vi "deserialize (HW-AIM).vi"(11 "data in":string[][](array[string])) -> (3 "hw configuration":T1[](array[typedef])=[{"terminalAddress"=[0]}, {"terminalAddress"=[1]}])   [LabVIEW 2020]
uses:
  _controls/aim1553_RT_list.ctl
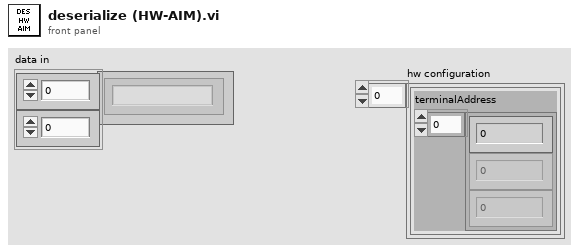
[diagram p1: front panel]
types:
  T1 = typedef "aim1553_RT_list.ctl" = cluster{"terminalAddress":i32[]}
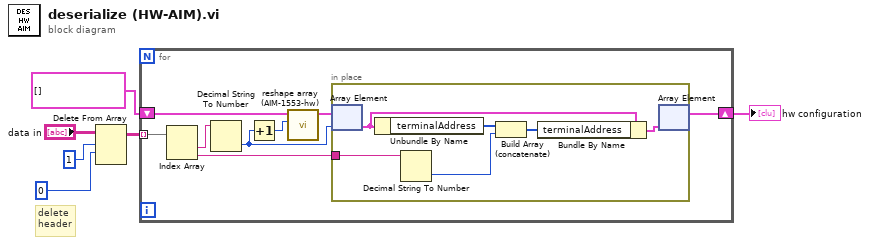
[diagram p0: block diagram]
diagram:
  # "delete\nheader"
  n1 = Delete From Array(array="data in", length=1, index (row)=0) -> (array with subset deleted=w3:string[][])  [unwired: 1 in, 1 out]
  n2 = for {
    tunnel: w3 -> [w14] mode=indexing
    shift-right: [w10] -> w1
    shift-left: T1[] [] ("hw configuration") -> [w9]
    n3 = Index Array(array=w14) -> (element #1=w12:string, element #2=w13:string)  [unwired: 2 in]
    n4 = Decimal String To Number(string=w12) -> (number=w11:i32)  [unwired: 2 in, 1 out]
    n5 = Increment(x=w11) -> (x+1=w8:i32)
    n6 = call "reshape array (AIM-1553-hw).vi"("size requested"=w8, "hw configuration in"=w9) -> ("hw configuration out"=w7:T1[])  [unwired: 9 in]
    n7 = in-place {
      in-place-border: w13 -> [w20]
      n8 = in-place-array #1(w7, w11) -> (w17:T1)
      n9 = Unbundle By Name(w17) -> ("terminalAddress"=w19:i32[])
      n10 = Decimal String To Number(string=w20) -> (number=w18:i32)  [unwired: 2 in, 1 out]
      n11 = Build Array (concatenate)(w19, w18) -> (w16:i32[])
      n12 = Bundle By Name(cluster=w17, "terminalAddress"=w16) -> (w15:T1)
      n13 = in-place-array #1(w15) -> (w10:T1[])  [unwired: 1 out]
    }
  }
  "hw configuration" <- w1
